vi "iRobot Sensor Stream Read (all sensors).vi"(8 "error in":errorcluster, 11 "UART port in":T9) -> (0 "error out":errorcluster, 1 "sensors":T1 {"Infrared" format="%02x"}, 2 "Packet Found?":bool, 3 "UART port out":T9)   [LabVIEW 2010]
doc: "Reads data from the UART serial port and updates sensors when packets are available.\n\nThis VI assumes that the robot is streaming all sensor data (sensor group 6).\n\nThis VI accumulates distance and angle whenever a new packet is received. The sensor components for distance and angle represent the accumulated amounts over the duration of the application execution. While this simplifies most code, which depends on how far the robot has moved, the developer must take account for rollover of signed 32-bit integers if the application has a long running time.\n\nNote that accumulated distance and angle tend to be extremeley inaccurate, since the iRobot looses fractional components of each when it sends a sensor update, and updates are sent at a high rate, resulting in significant roundoff error.\n\nThis VI reads from, but does not write to, the serial port."
uses:
  UART/UART Port Type.ctl
  Sensor Controls/iRobot Sensor Group 6.ctl
  Sensor Controls/iRobot Bumps + Wheel Drops.ctl
  Sensor Controls/iRobot Low-Side Driver + Wheel Overcurrent.ctl
  Sensor Controls/iRobot Buttons.ctl
  Sensor Controls/iRobot Charging State.ctl
  Sensor Controls/iRobot Cargo Bay Digital Inputs.ctl
  Sensor Controls/iRobot Charging Sources Available.ctl
  Sensor Controls/iRobot OI Mode.ctl
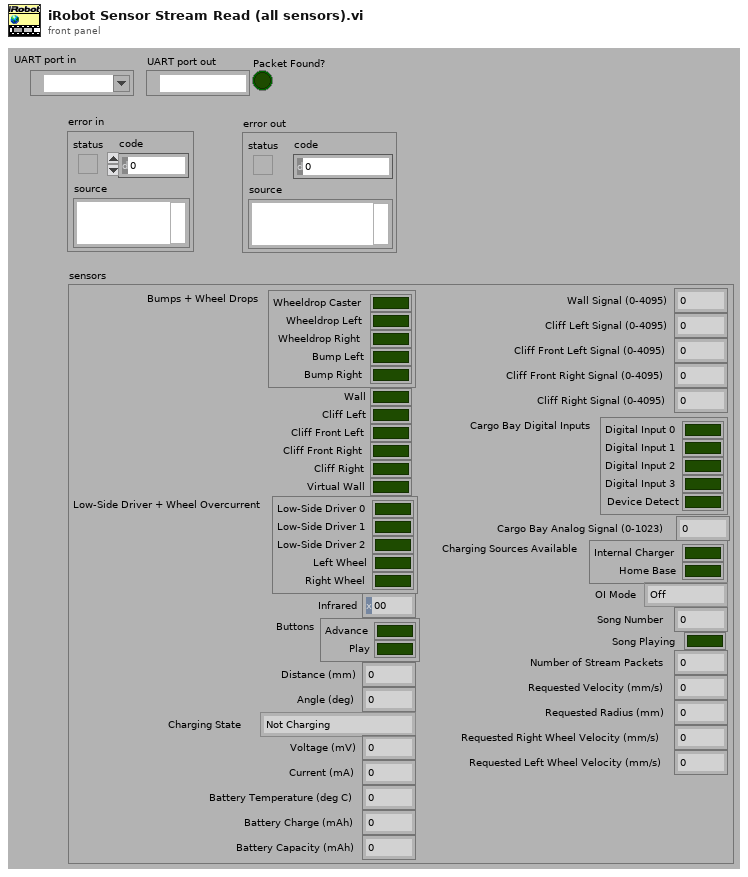
[diagram p1: front panel]
types:
  T1 = typedef "iRobot Sensor Group 6.ctl" = cluster{"Bumps + Wheel Drops":T2, "Wall":bool, "Cliff Left":bool, "Cliff Front Left":bool, "Cliff Front Right":bool, "Cliff Right":bool, "Virtual Wall":bool, "Low-Side Driver + Wheel Overcurrent":T3, "Infrared":u8, "Buttons":T4, "Distance (mm)":i32, "Angle (deg)":i32, "Charging State":T5, "Voltage (mV)":u16, "Current (mA)":i16, "Battery Temperature (deg C)":i8, "Battery Charge (mAh)":u16, "Battery Capacity (mAh)":u16, "Wall Signal (0-4095)":u16, "Cliff Left Signal (0-4095)":u16, "Cliff Front Left Signal (0-4095)":u16, "Cliff Front Right Signal (0-4095)":u16, "Cliff Right Signal (0-4095)":u16, "Cargo Bay Digital Inputs":T6, "Cargo Bay Analog Signal (0-1023)":u16, "Charging Sources Available":T7, "OI Mode":T8, "Song Number":u8, "Song Playing":bool, "Number of Stream Packets":u8, "Requested Velocity (mm/s)":u8, "Requested Radius (mm)":u8, "Requested Right Wheel Velocity (mm/s)":u8, "Requested Left Wheel Velocity (mm/s)":u8}
  T2 = typedef "iRobot Bumps + Wheel Drops.ctl" = cluster{"Wheeldrop Caster":bool, "Wheeldrop Left":bool, "Wheeldrop Right":bool, "Bump Left":bool, "Bump Right":bool}
  T3 = typedef "iRobot Low-Side Driver + Wheel Overcurrent.ctl" = cluster{"Low-Side Driver 0":bool, "Low-Side Driver 1":bool, "Low-Side Driver 2":bool, "Left Wheel":bool, "Right Wheel":bool}
  T4 = typedef "iRobot Buttons.ctl" = cluster{"Advance":bool, "Play":bool}
  T5 = typedef "iRobot Charging State.ctl" = enum16{"Not Charging", "Reconditioning Charging", "Full Charging", "Trickle Charging", "Waiting", "Charging Fault Condition"}
  T6 = typedef "iRobot Cargo Bay Digital Inputs.ctl" = cluster{"Digital Input 0":bool, "Digital Input 1":bool, "Digital Input 2":bool, "Digital Input 3":bool, "Device Detect":bool}
  T7 = typedef "iRobot Charging Sources Available.ctl" = cluster{"Internal Charger":bool, "Home Base":bool}
  T8 = typedef "iRobot OI Mode.ctl" = enum16{"Off", "Passive", "Safe", "Full"}
  T9 = typedef "UART Port Type.ctl" = refnum<visa-resource-name>
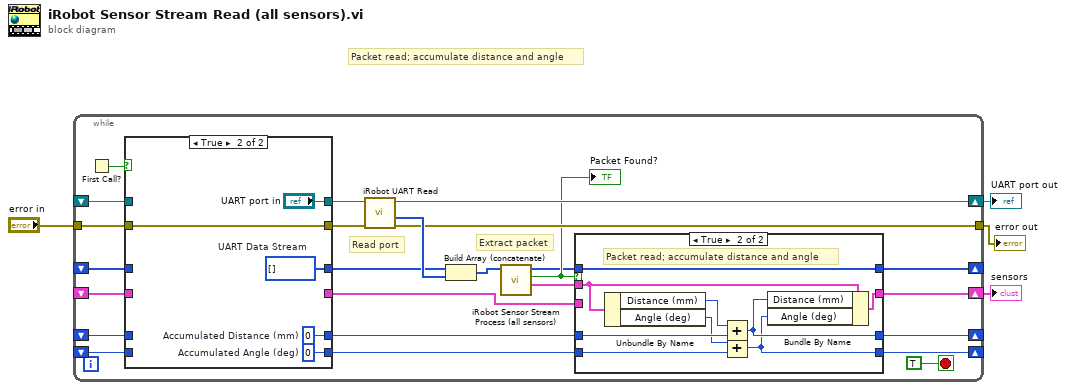
[diagram p0: block diagram]
diagram:
  # "Packet read; accumulate distance and angle"
  n1 = while {
    shift-right: [w22] -> w4
    shift-left: _ -> [w27]
    shift-right: [w6] -> _
    shift-left: _ -> [w25]
    shift-right: [w5] -> w3
    shift-left: _ -> [w20]
    tunnel: "error in" -> [w19]
    tunnel: [w17] -> w1
    shift-right: [w12] -> _
    shift-left: _ -> [w10]
    shift-right: [w11] -> _
    shift-left: _ -> [w9]
    stop <- TRUE stop-if-true
    # "Extract packet"
    # "Read port"
    n2 = First Call?() -> (First Call?: T/F=w29:bool)
    n3 = case shown="True" w29 {
      tunnel: [w47 "UART port in"] -> w26
      tunnel: w27 -> [w47 _]
      tunnel: w25 -> [w48 _]
      tunnel: [w48 w53] -> w23
      tunnel: w20 -> [w46 _]
      tunnel: [w46 _] -> w8
      tunnel: w19 -> [w45 w49]
      tunnel: [w45 w49] -> w18
      tunnel: [w44 w52] -> w14
      tunnel: [w43 w51] -> w13
      tunnel: w10 -> [w44 _]
      tunnel: w9 -> [w43 _]
      frame False {
        # "Stream already initialized."
      }
      frame True {
        w51 = 0  # Accumulated Angle (deg)
        w52 = 0  # Accumulated Distance (mm)
        w53 = u8[] []  # UART Data Stream
      }
    }
    n4 = call "iRobot UART Read.vi"("error in"=w18, "UART port in"=w26) -> ("error out"=w17:errorcluster, "data"=w24:u8[], "UART port out"=w22:T9)  [unwired: 7 in]
    n5 = Build Array (concatenate)(w23, w24) -> (w21:u8[])
    n6 = call "iRobot Sensor Stream Process (all sensors).vi"("stream in"=w21) -> ("sensors"=w15:T1, "Packet Found?"=w16:bool, "stream out"=w7:u8[])  [unwired: 8 in]
    "Packet Found?" <- w16
    n7 = case shown="True" w16 {
      tunnel: w15 -> [_ w34]
      tunnel: w14 -> [w33 w41]
      tunnel: w13 -> [w32 w39]
      tunnel: [w33 w37] -> w12
      tunnel: [w32 w36] -> w11
      tunnel: w8 -> [w30 _]
      tunnel: [w31 w42] -> w6
      tunnel: w7 -> [w31 w42]
      tunnel: [w30 w35] -> w5
      frame False {
        # "No packet read; retain previous sensors.\naccumulated distance, and accumulated  angle"
      }
      frame True {
        # "Packet read; accumulate distance and angle"
        n8 = Unbundle By Name(w34) -> ("Distance (mm)"=w40:i32, "Angle (deg)"=w38:i32)
        n9 = Add(x=w40, y=w41) -> (x+y=w37:i32)
        n10 = Add(x=w38, y=w39) -> (x+y=w36:i32)
        n11 = Bundle By Name(cluster=w34, "Distance (mm)"=w37, "Angle (deg)"=w36) -> (w35:T1)
      }
    }
  }
  "UART port out" <- w4
  "sensors" <- w3
  "error out" <- w1
